vi "update AlarmCode XML.vi"(8 "error in (no error)":errorcluster) -> (0 "error out":errorcluster)   [LabVIEW 2022 SP3, in "opSignIn.lvlib"]
uses:
  opSignIn.lvlib
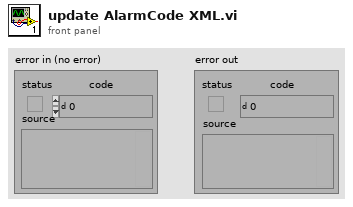
[diagram p1: front panel]
types:
  T1 = cluster{"url":string, "loginTokenRequest":cluster{"clientId":string, "clientSecret":string, "grantType":string, "password":string, "scope":string, "userName":string, "userType":string}, "自动获取MN":bool}
  T2 = cluster{"code":string, "message":string, "timestamp":u64, "data":cluster{"bearerType":string, "oauth2Type":string, "accessToken":string, "tokenType":string, "expiresIn":u64, "refreshToken":string, "scope":string[], "tokenDetail":cluster{"dataSource":string, "username":string, "userId":string, "userType":string, "enabled":bool, "accountNonExpired":bool, "credentialsNonExpired":bool, "accountNonLocked":bool}}, "success":bool}
  T3 = typedef "opSignIn.lvlib/报警格式.ctl" = cluster{"data":T4[]}
  T4 = typedef "opSignIn.lvlib/元素.ctl" = cluster{"id":string, "componentParentId":string, "componentParentName":string, "componentParentPath":string, "componentId":string, "componentName":string, "faultName":string, "equipVersion":string, "alarmCode":string, "supportAlarm":bool, "ipcAlarmCode":string, "sort":dbl, "solutionList":cluster{"id":string, "faultId":string, "reason":string, "dataPhenomenon":string, "analysis":string, "solution":string}[]}
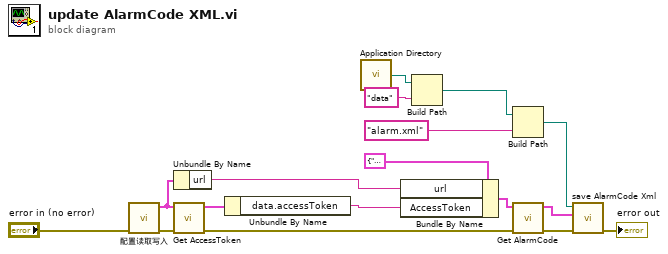
[diagram p0: block diagram]
diagram:
  n1 = call "配置读取写入.vi"("error in (no error)"="error in (no error)") -> ("error out"=w16:errorcluster, "配置输出"=w14:T1)  [unwired: 9 in]
  n2 = Unbundle By Name(w14) -> ("url"=w13:string)
  n3 = call "Get AccessToken.vi"("error in (no error)"=w16, "配置"=w14) -> ("error out"=w9:errorcluster, "response"=w12:T2)  [unwired: 8 in]
  n4 = Unbundle By Name(w12) -> ("data.accessToken"=w11:string)
  n5 = call <vilib>:"Application Directory.vi"() -> ("Application Directory"=w6:path)
  n6 = Bundle By Name(cluster=cluster{"url":string, "AccessToken":string} {"url"="http://data.watersystem.com.cn:50040", "AccessToken"="equip&GbbVkGRBUSaIfhTSjiolTAP8QMM"} ("Para"), "url"=w13, "AccessToken"=w11) -> (w10:cluster{"url":string, "AccessToken":string})
  n7 = Build Path(base path=w6, name or relative path="data" ("名称或相对路径")) -> (appended path=w4:path)
  n8 = Build Path(base path=w4, name or relative path="alarm.xml" ("default name")) -> (appended path=w2:path)
  n9 = call "Get AlarmCode.vi"("error in (no error)"=w9, "Para"=w10) -> ("error out"=w1:errorcluster, "project"=w7:T3)  [unwired: 8 in]
  n10 = call "save AlarmCode Xml.vi"("error in (no error)"=w1, "project"=w7, "XML File Path"=w2) -> ("error out"=→"error out":errorcluster)  [unwired: 8 in]
